vi "example call ref cancel.vi"() -> ()   [LabVIEW 2013]
uses:
  result/result.lvclass
  dispatcher/pool sizes.ctl
  dispatcher/execution system.ctl
  standard tokens/cancel token/cancel token.lvclass
  result/result.lvclass/result.ctl
  result/get data.vi
  result/get error.vi
  result/get generating action.vi
  result/get owning task.vi
  result/get subresults.vi
  dispatcher/thread pool.lvclass
  standard reporters/event reporter/event reporter.lvclass
  standard tasks/function task/function task.lvclass
  standard action/call by reference action/call by reference action.lvclass
panel:
  out "time to cancel":u32
  out "subresults":refnum<class "result.lvclass">[](array[class])
  out "owning task":string
  out "generating action":string
  out "error":errorcluster
  out "data":variant
  out "Time":u32
  out "result":refnum<class "result.lvclass">
  out "error out":errorcluster
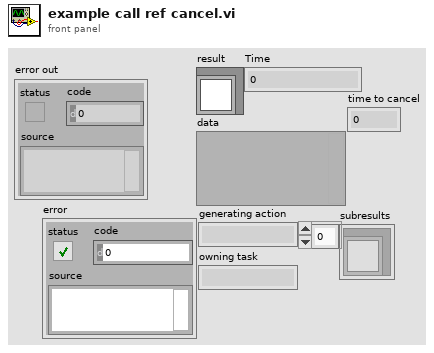
[diagram p1: front panel]
types:
  T1 = typedef "thread pool.lvclass/execution system.ctl" = enum32{"user interface", "standard", "instrument i/o", "data acquisition", "other 1", "other 2"}
  T2 = typedef "thread pool.lvclass/pool sizes.ctl" = cluster{"UI thread":u8, "standard":u8, "instrument I/O":u8, "data acquisition":u8, "other 1":u8, "other 2":u8}
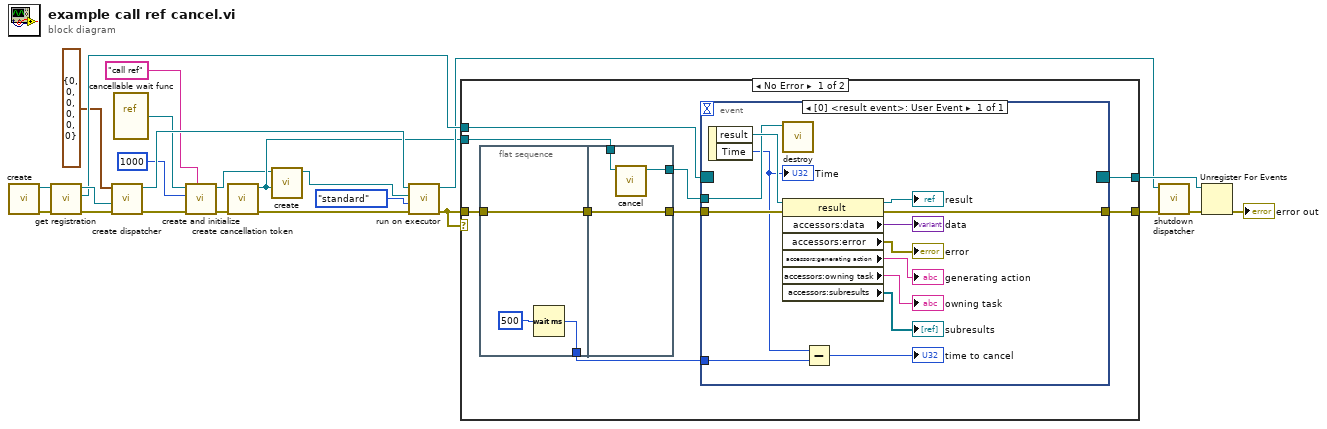
[diagram p0: block diagram]
diagram:
  n1 = call "create.vi"() -> ("error out"=w21:errorcluster, "event reporter out"=w22:refnum<class "event reporter.lvclass">)  [unwired: 10 in]
  n2 = call "get registration.vi"("error in"=w21, "event reporter in"=w22) -> ("error out"=w19:errorcluster, "result registration"=w18:refnum<event-registration>, "event reporter out"=w20:refnum<class "event reporter.lvclass">)  [unwired: 7 in]
  n3 = call "create dispatcher.vi"("error in"=w19, "default reporter"=w20, "initial pool sizes"=T2 {"UI thread"=0, "standard"=0, "instrument I/O"=0, "data acquisition"=0, "other 1"=0, "other 2"=0}) -> ("error out"=w3:errorcluster, "dispatcher"=w23:refnum<data-value>)  [unwired: 7 in]
  n4 = vi-ref "cancellable wait func.vi"() -> (w6:refnum<vi>)
  n5 = call "create and initialize.vi"("action name"="call ref", "error in"=w3, "parameters"=1000, "function"=w6) -> ("error out"=w2:errorcluster, "call by reference action"=w1:refnum<class "call by reference action.lvclass">)  [unwired: 6 in]
  n6 = call "create cancellation token.vi"("error in"=w2) -> ("error out"=w8:errorcluster, "cancel token out"=w7:refnum<class "cancel token.lvclass">)  [unwired: 9 in]
  n7 = call "create.vi"("task token"=w7, "action"=w1) -> ("function task out"=w12:refnum<class "function task.lvclass">)  [unwired: 9 in]
  n8 = call "run on executor.vi"("error in"=w8, "execution system"=execution_system."standard", "task"=w12, "dispatcher"=w23) -> ("error out"=w11:errorcluster, "dispatcher out"=w16:refnum<data-value>)  [unwired: 6 in]
  n9 = case shown="No Error" w11 {
    tunnel: w18 -> [w32 w53]
    tunnel: [w31 w53] -> w17
    tunnel: [w30 w52] -> w13
    tunnel: w11 -> [w28 w52]
    tunnel: w7 -> [w26 _]
    frame No Error {
      n10 = flat-sequence {
        tunnel: w28 -> [w35]
        tunnel: [w35] -> w27
        tunnel: [w33] -> w24
        tunnel: [w38] -> w29
        tunnel: w27 -> [w38]
        tunnel: w26 -> [w37]
        tunnel: [w36] -> w25
        frame #0 {
          n11 = Wait (ms)(milliseconds to wait=u32 500) -> (millisecond timer value=w33:u32)
        }
        frame #1 {
          n12 = call-dynamic "cancel.vi"("cancel token in"=w37) -> ("cancel token out"=w36:refnum<class "cancel token.lvclass">)  [unwired: 9 in, 1 out]
        }
      }
      n13 = event shown="[0] <result event>: User Event" {
        selector: w32 -> [_]
        dyn-events: [_] -> w31
        timeout: _ -> [_]
        tunnel: [w50] -> w30
        tunnel: w29 -> [w51]
        tunnel: w25 -> [w42]
        tunnel: w24 -> [w40]
        event User Event {
          n14 = event-data() -> ("result"=w49:refnum<class "result.lvclass">, "Time"=w41:u32)  [unwired: 1 in]
          "Time" <- w41
          n15 = call-dynamic "destroy.vi"("task token in"=w42) -> ()  [unwired: 10 in, 1 out]
          n16 = property class="result"(reference=w49, error in=w51) -> (reference out=→"result":refnum<class "result.lvclass">, error out=w50:errorcluster, "accessors:data"=→"data":variant, "accessors:error"=→"error":errorcluster, "accessors:generating action"=→"generating action":string, "accessors:owning task"=→"owning task":string, "accessors:subresults"=→"subresults":refnum<class "result.lvclass">[])
          n17 = Subtract(x=w41, y=w40) -> (x-y=→"time to cancel":u32)
        }
      }
    }
    frame Error {
    }
  }
  n18 = call "shutdown dispatcher.vi"("error in"=w13, "dispatcher"=w16) -> ("error out"=w15:errorcluster)  [unwired: 9 in]
  n19 = Unregister For Events(event registration refnum=w17, error in=w15) -> (error out=→"error out":errorcluster)
